vi "test dummy.vi"() -> ()   [LabVIEW 2020, in "Method Generation.lvlib" / "Getter Generator.lvclass"]
uses:
  Getter Generator.lvclass
  Framework/Process/Process.lvclass
panel:
  in  "Message Data":variant
  in  "Message":string
  out "Process Out":refnum<class "Process.lvclass">
  in  "Process In":refnum<class "Process.lvclass">
  out "error out":errorcluster
  in  "error in (no error)":errorcluster
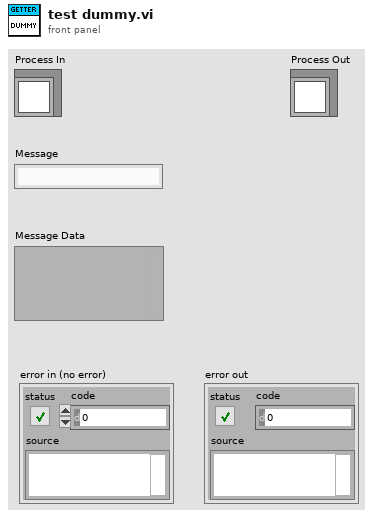
[diagram p1: front panel]
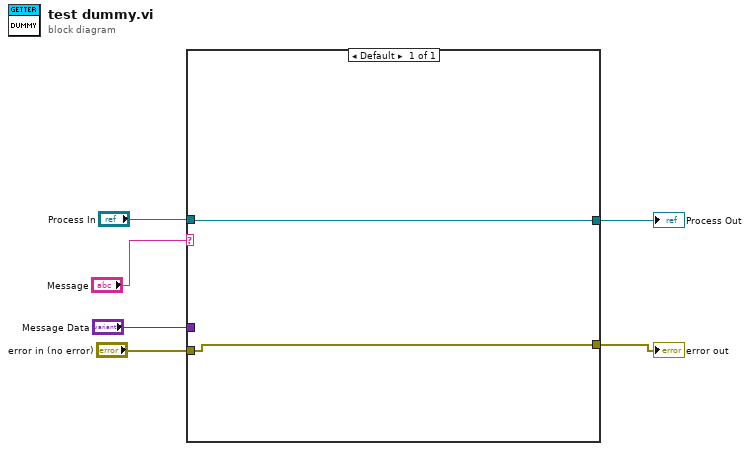
[diagram p0: block diagram]
diagram:
  n1 = case shown="Default" "Message" {
    tunnel: [w7] -> w6
    tunnel: "Process In" -> [w7]
    tunnel: [w8] -> w4
    tunnel: "error in (no error)" -> [w8]
    tunnel: "Message Data" -> [_]
    frame Default {
    }
  }
  "error out" <- w4
  "Process Out" <- w6
